vi "Constructor.vi"(8 "error in (no error)":errorcluster, 11 "Top Level Diagram":refnum<vi>) -> (0 "error out":errorcluster, 3 "Block Diagram":refnum<class "Block Diagram.lvclass">)   [LabVIEW 2015, in "Block Diagram.lvclass"]
uses:
  Block Diagram.lvclass
  Initial Sequence/Initial Sequence.lvclass
  DMA Loop/DMA Loop.lvclass
  Analog Input Loop/Analog Input Loop.lvclass
  Analog Output Loop/Analog Output Loop.lvclass
  Digital High Speed Loop/Digital High Speed Loop.lvclass
  Digital Slow Speed Loop/Digital Slow Speed Loop.lvclass
  Block Diagram.lvclass/Block Diagram.ctl
  Module Loop/Module Loop.lvclass
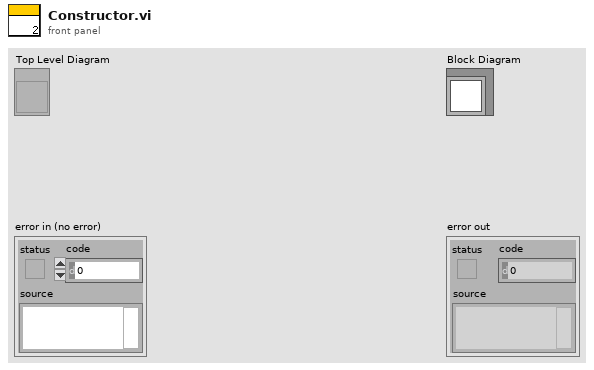
[diagram p1: front panel]
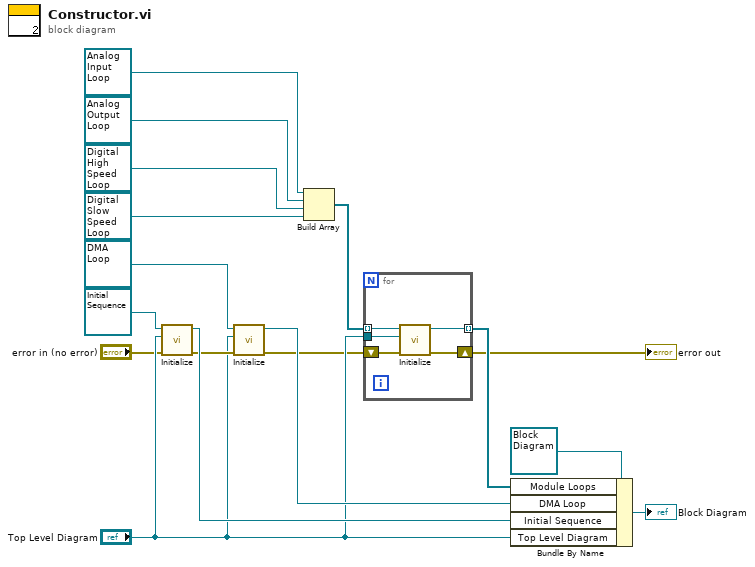
[diagram p0: block diagram]
diagram:
  n1 = call-dynamic "Initialize.vi"("error in (no error)"="error in (no error)", "Top Level Diagram"="Top Level Diagram", "Initial Sequence in"=refnum<class "Initial Sequence.lvclass"> refnum ("Initial Sequence.lvclass")) -> ("error out"=w12:errorcluster, "Initial Sequence out"=w13:refnum<class "Initial Sequence.lvclass">)  [unwired: 7 in]
  n2 = call-dynamic "Initialize.vi"("error in (no error)"=w12, "Top Level Diagram"="Top Level Diagram", "DMA Loop in"=refnum<class "DMA Loop.lvclass"> refnum ("DMA Loop.lvclass")) -> ("error out"=w2:errorcluster, "DMA Loop out"=w14:refnum<class "DMA Loop.lvclass">)  [unwired: 7 in]
  n3 = Build Array(refnum<class "Analog Input Loop.lvclass"> refnum ("Analog Input Loop.lvclass"), refnum<class "Analog Output Loop.lvclass"> refnum ("Analog Output Loop.lvclass"), refnum<class "Digital High Speed Loop.lvclass"> refnum ("Digital High Speed Loop.lvclass"), refnum<class "Digital Slow Speed Loop.lvclass"> refnum ("Digital Slow Speed Loop.lvclass")) -> (w3:refnum<class "Module Loop.lvclass">[])
  n4 = for {
    tunnel: "Top Level Diagram" -> [w20]
    shift-right: [w22] -> w1
    shift-left: w2 -> [w21]
    tunnel: w3 -> [w19] mode=indexing
    tunnel: [w18] -> w4 mode=indexing
    n5 = call-dynamic "Initialize.vi"("error in (no error)"=w21, "Top Level Diagram"=w20, "IO Loop in"=w19) -> ("error out"=w22:errorcluster, "IO Loop out"=w18:refnum<class "Module Loop.lvclass">)  [unwired: 7 in]
  }
  "error out" <- w1
  n6 = Bundle By Name(cluster=refnum<class "Block Diagram.lvclass"> refnum ("Block Diagram.lvclass"), "Module Loops"=w4, "DMA Loop"=w14, "Initial Sequence"=w13, "Top Level Diagram"="Top Level Diagram") -> (→"Block Diagram":refnum<class "Block Diagram.lvclass">)
